vi "Read_image.vi"(10 "Type":string="_pinout.png", 11 "ProductNum":u32) -> ()   [LabVIEW 2017, in "ALMA_10201-10401_O2SensorSim System Explorer.lvlib"]
uses:
  ALMA_10201-10401_O2SensorSim System Explorer.lvlib
  <vilib>/Utility/sysdir.llb/System Directory Type.ctl
  <vilib>/Utility/miscctls.llb/LVBoundsTypeDef.ctl
panel:
  out "2D Picture":picture
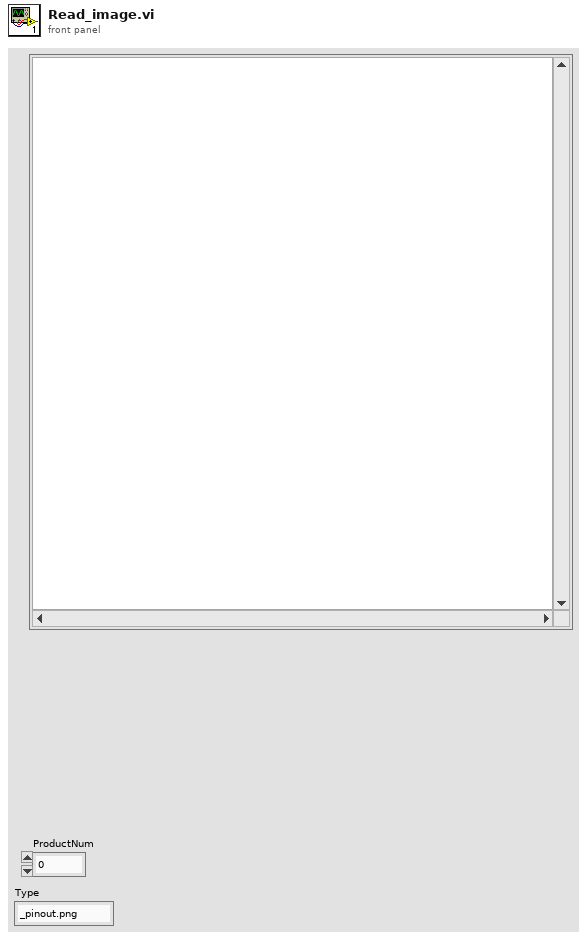
[diagram p1: front panel]
types:
  T1 = typedef "System Directory Type.ctl" = i32
  T2 = typedef "imagedata.ctl" = cluster{"image type":i32, "image depth":i32, "image":u8[], "mask":u8[], "colors":u32[], "Rectangle":cluster{"left":i16, "top":i16, "right":i16, "bottom":i16}}
  T3 = typedef "LVBoundsTypeDef.ctl" = cluster{"Width":u32, "Height":u32}
  T4 = cluster{"left":i16, "top":i16, "right":i16, "bottom":i16}
  T5 = typedef "LVRectTypeDef.ctl" = cluster{"Left":i16, "Top":i16, "Right":i16, "Bottom":i16}
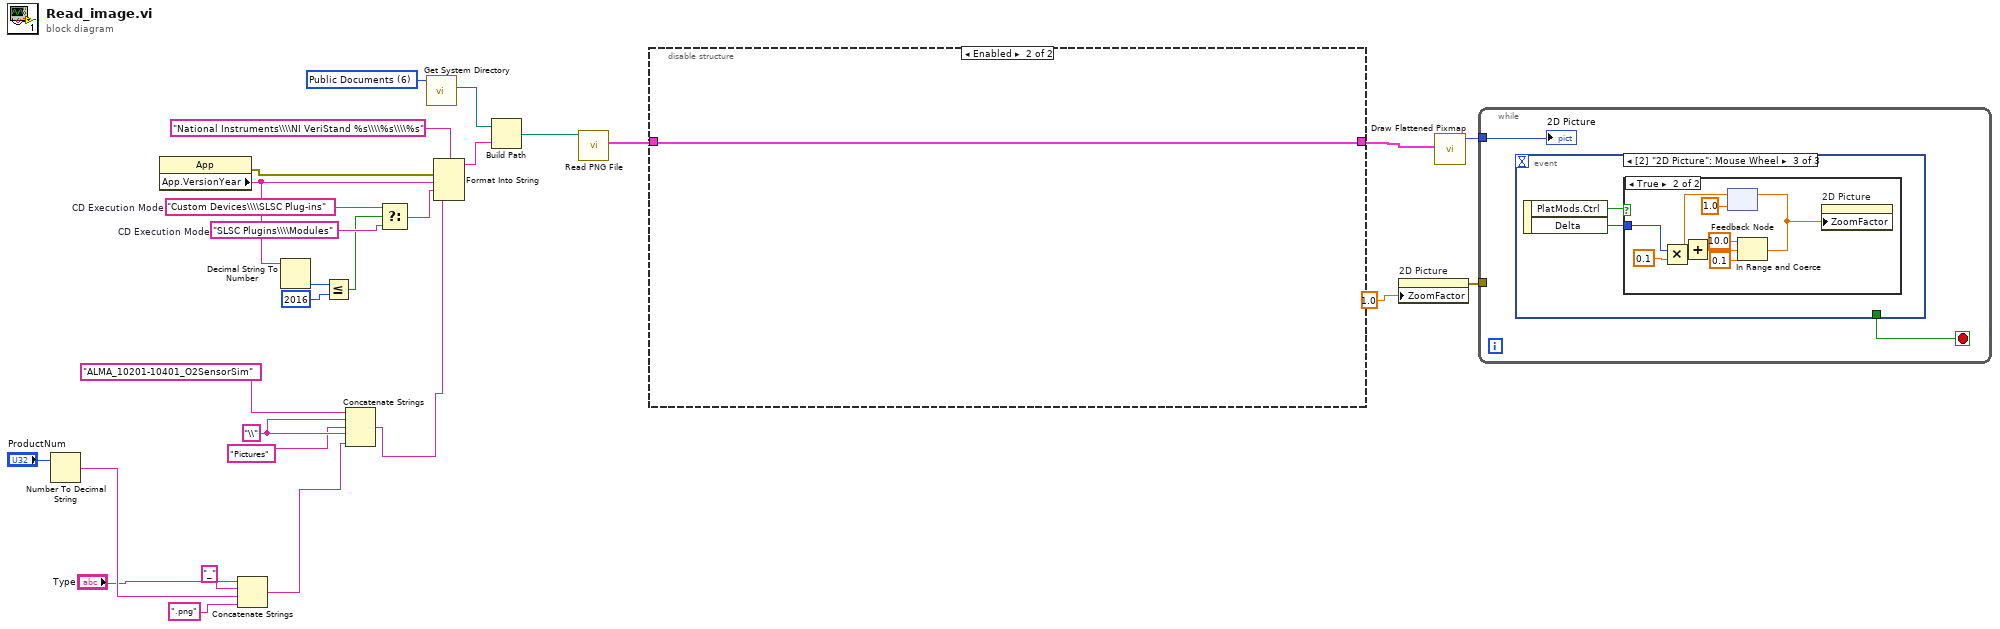
[diagram p0: block diagram]
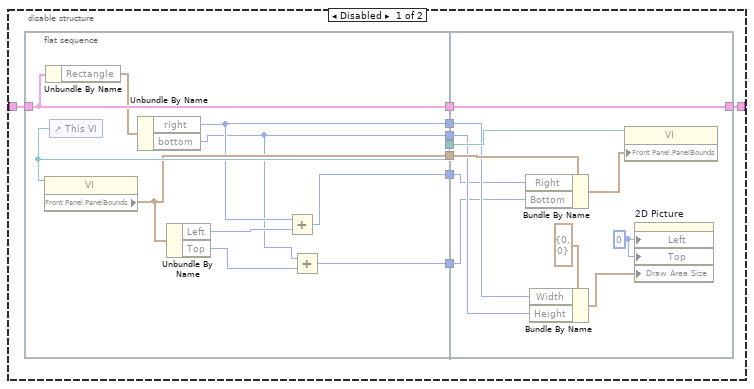
[diagram p2: hidden frame]
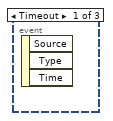
[diagram p3: hidden frame]
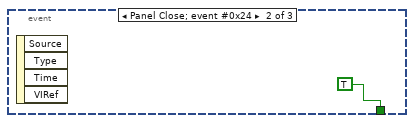
[diagram p4: hidden frame]
diagram:
  w7 = "\\" ("string")
  w26 = "SLSC Plugins\\\\Modules"  # CD Execution Mode
  w27 = "Custom Devices\\\\SLSC Plug-ins"  # CD Execution Mode
  w18 = T1 6 items=["User Home"=0, "User Desktop"=1, "User Documents"=2, "User Application Data"=3, "User Preferences"=4, "User Temporary"=5, "Public Documents"=6, "Public Application Data"=7, "Public Preferences"=8, "Public Cache"=13, "System Core Libraries"=9, "System Installed Libraries"=10, "Application Files"=11, "Boot Volume Root"=12] ("system directory type")
  n1 = Number To Decimal String(number="ProductNum") -> (decimal integer string=w12:string)  [unwired: 1 in]
  n2 = property class="App"() -> (error out=w19:errorcluster, "App.VersionYear"=w21:string)  [unwired: 2 in, 1 out]
  n3 = Concatenate Strings("Type", "_" ("string"), w12, ".png" ("string")) -> (w1:string)
  n4 = Decimal String To Number(string=w21) -> (number=w22:i32)  [unwired: 2 in, 1 out]
  n5 = Less Or Equal?(x=w22, y=2016) -> (x <= y?=w25:bool)
  n6 = Concatenate Strings("ALMA_10201-10401_O2SensorSim" ("string"), w7, "Pictures" ("string"), w7, w1) -> (w13:string)
  n7 = Select(t=w27, s=w25, f=w26) -> (s? t:f=w24:string)
  n8 = call <vilib>:"Get System Directory.vi"("system directory type"=w18) -> ("system directory"=w17:path)  [unwired: 10 in]
  n9 = Format Into String(format string="National Instruments\\\\NI VeriStand %s\\\\%s\\\\%s" ("name or relative path"), error in=w19, w21, w24, w13) -> (resulting string=w16:string)  [unwired: 1 in, 1 out]
  n10 = Build Path(base path=w17, name or relative path=w16) -> (appended path=w9:path)
  n11 = call <vilib>:"Read PNG File.vi"("path to PNG file"=w9) -> ("image data"=w10:T2)  [unwired: 8 in, 2 out]
  n12 = disable-structure shown="Enabled" {
    disable-tunnel: w10 -> [w30 w59]
    disable-tunnel: [w29 w59] -> w2
    frame Disabled {
      n13 = flat-sequence {
        tunnel: w30 -> [w47]
        tunnel: [w47] -> w37
        tunnel: [w46] -> w36
        tunnel: [w44] -> w35
        tunnel: [w42] -> w34
        tunnel: [w41] -> w33
        tunnel: [w40] -> w32
        tunnel: [w39] -> w31
        tunnel: w37 -> [w48]
        tunnel: w36 -> [w58]
        tunnel: w35 -> [w57]
        tunnel: w34 -> [w50]
        tunnel: w33 -> [w49]
        tunnel: w32 -> [w52]
        tunnel: w31 -> [w51]
        tunnel: [w48] -> w29
        frame #0 {
          n14 = Unbundle By Name(w47) -> ("Rectangle"=w45:T4)
          n15 = control-ref of="This VI"() -> (w46:refnum<vi>)
          n16 = property class="VI"(reference=w46) -> ("Front Panel.PanelBounds"=w44:T5)  [unwired: 1 in, 2 out]
          n17 = Unbundle By Name(w45) -> ("right"=w40:i16, "bottom"=w39:i16)
          n18 = Unbundle By Name(w44) -> ("Left"=w43:i16, "Top"=w38:i16)
          n19 = Add(x=w40, y=w43) -> (x+y=w42:i16)
          n20 = Add(x=w39, y=w38) -> (x+y=w41:i16)
        }
        frame #1 {
          w55 = i16 0 ("Origin:Left")
          n21 = Bundle By Name(cluster=w57, "Right"=w50, "Bottom"=w49) -> (w56:T5)
          n22 = Bundle By Name(cluster=T3 {"Width"=0, "Height"=0} ("Draw Area Size"), "Width"=w52, "Height"=w51) -> (w53:T3)
          n23 = property class="VI"(reference=w58, "Front Panel.PanelBounds"=w56) -> ()  [unwired: 1 in, 2 out]
          n24 = property on="2D Picture" class="Pict"("Left"=w55, "Top"=w55, "Draw Area Size"=w53) -> ()  [unwired: 2 in, 2 out]
        }
      }
    }
    frame Enabled {
    }
  }
  n25 = property on="2D Picture" class="Pict"("ZoomFactor"=sgl 1.0 ("Zoom Factor")) -> (error out=w5:errorcluster)  [unwired: 2 in, 1 out]
  n26 = call <vilib>:"Draw Flattened Pixmap.vi"("image data"=w2) -> ("new picture"=w4:picture)  [unwired: 8 in]
  n27 = while {
    tunnel: w4 -> [w61]
    tunnel: w5 -> [_]
    stop <- w60 stop-if-true
    n28 = event shown="[2] \"2D Picture\": Mouse Wheel" {
      selector: _ -> [_ _ _]
      dyn-events: _ -> [_ _ _]
      timeout: _ -> [_ _ _]
      tunnel: [_ TRUE _] -> w60
      event Timeout {
        n29 = event-data() -> ()  [unwired: 1 in, 3 out]
      }
      event Panel Close; event #0x24 {
        n30 = event-data() -> ()  [unwired: 1 in, 4 out]
      }
      event "2D Picture": Mouse Wheel {
        n31 = event-data() -> ("PlatMods.Ctrl"=w63:bool, "Delta"=w64:i32)  [unwired: 1 in]
        n32 = case shown="True" w63 {
          tunnel: w64 -> [_ w66]
          frame False {
          }
          frame True {
            n33 = Multiply(x=w66, y=0.1) -> (x*y=w72:dbl)
            n34 = feedback #1(1.0 ("upper limit")) -> (w70:dbl)
            n35 = Add(x=w70, y=w72) -> (x+y=w71:dbl)
            n36 = In Range and Coerce(upper limit=10.0, x=w71, lower limit=0.1) -> (coerced(x)=w65:dbl)  [unwired: 1 out]
            n37 = feedback-in #1(w65) -> ()
            n38 = property on="2D Picture" class="Pict"("ZoomFactor"=w65) -> ()  [unwired: 2 in, 2 out]
          }
        }
      }
    }
    "2D Picture" <- w61
  }
